vi "Rack-Init.vi"(8 "error in (no error)":errorcluster) -> (0 "error out":errorcluster, 2 "OutputRequest\nevent ref":T1)   [LabVIEW 2015]
doc: "Initializes the Rack subsystems. Call this before doing anything else.\n\nIt resets the port reservation system (which needs to be done before initializing devices) and creates the OutputRequest user event refnum."
uses:
  Typedefs/OutputRequest refnum.ctl
  Typedefs/OutputRequest.ctl
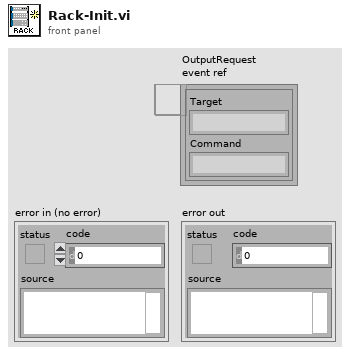
[diagram p1: front panel]
types:
  T1 = typedef "OutputRequest refnum.ctl" = refnum<user-event>
  T2 = typedef "OutputRequest.ctl" = cluster{"Target":string, "Command":string}
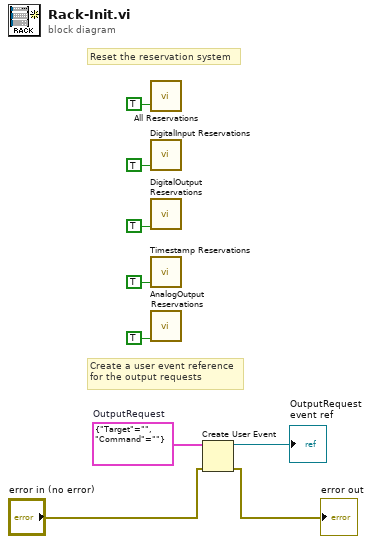
[diagram p0: block diagram]
diagram:
  w5 = T2 {"Target"="", "Command"=""}  # OutputRequest
  # "Create a user event reference\nfor the output requests"
  # "Reset the reservation system"
  n1 = call "All Reservations.vi"("Reset"=TRUE) -> ()  [unwired: 1 in, 2 out]
  n2 = call "DigitalInput Reservations.vi"("Reset"=TRUE) -> ()  [unwired: 2 in, 3 out]
  n3 = call "DigitalOutput Reservations.vi"("Reset"=TRUE) -> ()  [unwired: 3 in, 4 out]
  n4 = call "Timestamp Reservations.vi"("Reset"=TRUE) -> ()  [unwired: 2 in, 3 out]
  n5 = call "AnalogOutput Reservations.vi"("Reset"=TRUE) -> ()  [unwired: 3 in, 4 out]
  n6 = Create User Event(user event datatype=w5, error in="error in (no error)") -> (user event=→"OutputRequest\nevent ref":refnum<user-event>, error out=→"error out":errorcluster)
